vi "TEMPERTAURE DISPLAY.vi"() -> ()   [LabVIEW 2015]
uses:
  <vilib>/Utility/file.llb/Write Delimited Spreadsheet (string).vi
panel:
  in  "Table":string[][](table)
  out "TEMP STATUS":string="OVER"
  out "time string":string
  out "date string":string
  in  "stop":bool
  out "Temp gone BELOW":bool
  out "Temperature gone ABOVE":bool
  in  "Temperature":dbl(slide) scale=0.0..50.0
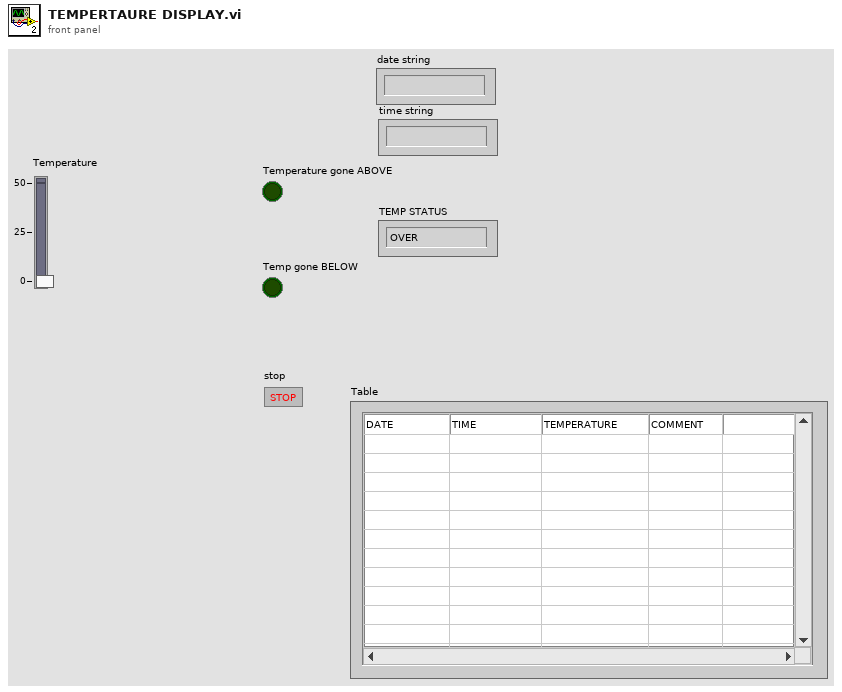
[diagram p1: front panel]
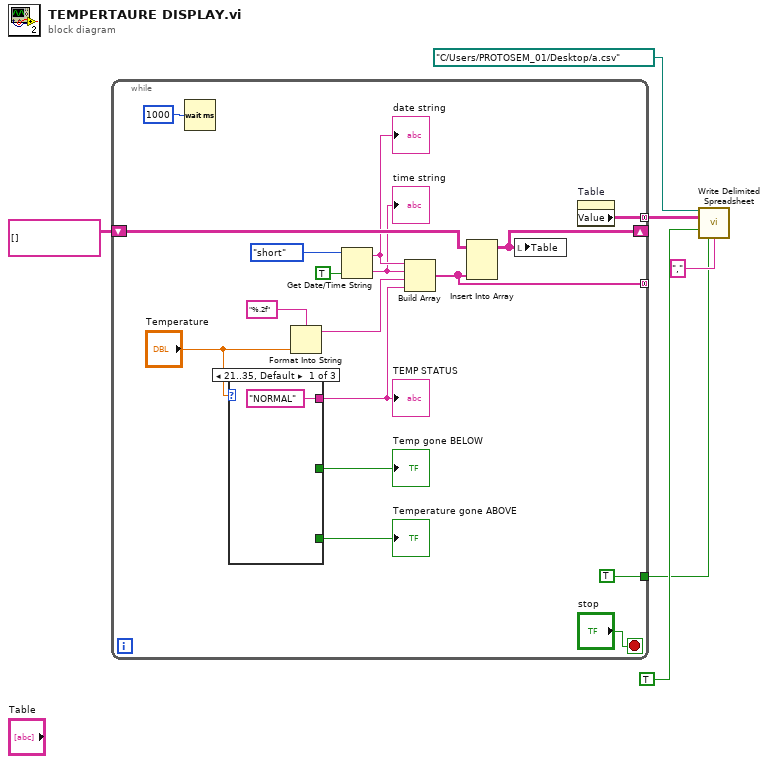
[diagram p0: block diagram]
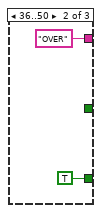
[diagram p2: hidden frame]
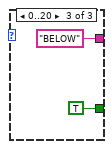
[diagram p3: hidden frame]
diagram:
  n1 = while {
    shift-right: [w10] -> _
    shift-left: string[][] [] -> [w17]
    tunnel: [w9] -> _ mode=concatenating
    tunnel: [TRUE ("transpose? (F)")] -> w2
    tunnel: [w7] -> w1 mode=concatenating
    stop <- "stop" stop-if-true
    n2 = Wait (ms)(milliseconds to wait=u32 1000) -> ()  [unwired: 1 out]
    n3 = case shown="21..35, Default" "Temperature" {
      tunnel: [_ TRUE ("Temperature gone ABOVE") _] -> w21
      tunnel: [_ _ TRUE ("Temp gone ABOVE")] -> w20
      tunnel: ["NORMAL" "OVER" "BELOW"] -> w11
      frame 21..35, Default {
      }
      frame 36..50 {
      }
      frame 0..20 {
      }
    }
    "Temperature gone ABOVE" <- w21
    "Temp gone BELOW" <- w20
    "TEMP STATUS" <- w11
    n4 = Format Into String(format string="%.2f", "Temperature") -> (resulting string=w12:string)  [unwired: 2 in, 1 out]
    n5 = Get Date/Time String(date format (0)=enum16{"short", "long", "abbreviated"}."short", want seconds? (F)=TRUE) -> (date string=w16:string, time string=w15:string)  [unwired: 1 in]
    "date string" <- w16
    "time string" <- w15
    n6 = Build Array(w16, w15, w12, w11) -> (w9:string[])
    n7 = Insert Into Array(array=w17, new element=w9) -> (w10:string[][])  [unwired: 2 in]
    n8 = local write "Table"(w10) -> ()
    n9 = property on="Table" class="Tbl (strict)"() -> ("Value"=w7:string[][])  [unwired: 2 in, 2 out]
  }
  n10 = call-poly <vilib>:"Write Delimited Spreadsheet.vi"("file path (dialog if empty)"=path "C:/Users/PROTOSEM_01/Desktop/a.csv", "2D data"=w1, "append to file? (F)"=TRUE, "transpose? (F)"=w2, "delimiter (\\t)"="," ("delimiter (\\t)")) -> ()  [unwired: 9 in, 2 out]
